vi "J-Turn.vi"(6 "Synchronication":enum16{"Start", "Wait"}(ring), 7 "Description":string, 8 "Command Info In":T2, 9 "Path Data":T1=[{"Maneuver"=enum."MAX 90", "Rotation Direction"=enum."N/A"}, {"Maneuver"=enum."MAX 90", "Rotation Direction"=enum."N/A"}, {"Maneuver"=enum."MAX 90", "Rotation Direction"=enum."N/A"}], 10 "Angle boi":dbl, 11 "Left Setpoint (Power)":dbl) -> (0 "Command Info Out":T2)   [LabVIEW 2018]
doc: "This VI notifies the subsystem to the new setpoint."
uses:
  <vilib>/Rock Robotics/WPI/Framework/Command Status Info.ctl
  <vilib>/Rock Robotics/WPI/Framework/Completion Status.ctl
  <vilib>/Rock Robotics/WPI/Framework/Completion Notifier.ctl
  Support Code/Path Data.ctl
  Implementation/Drive Operations.ctl
  Implementation/Drive Setpoints.ctl
  Support Code/Availible Command systems for auto.ctl
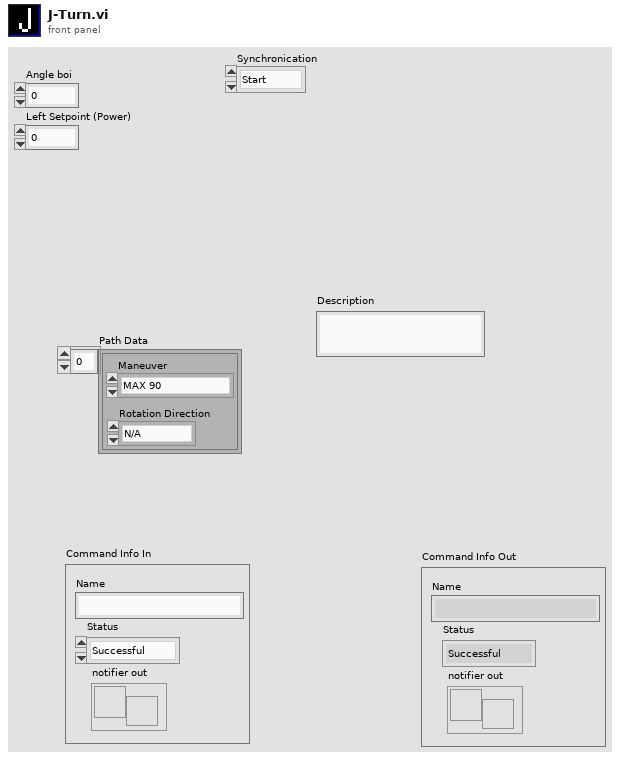
[diagram p1: front panel]
types:
  T1 = typedef "Path Data.ctl" = cluster{"Maneuver":enum16{"MAX 90", "MAX 180", "Turn to Home", "Turn to Rocket", "Auto-Align", "Turn to ..."}, "Rotation Direction":enum16{"N/A", "Right", "Left"}}[]
  T2 = typedef "Command Status Info.ctl" = cluster{"Name":string, "Status":T3, "notifier out":T4}
  T3 = typedef "Completion Status.ctl" = enum16{"Successful", "Aborted", "Incomplete"}
  T4 = typedef "Completion Notifier.ctl" = refnum<notifier>
  T5 = typedef "Drive Operations.ctl" = enum16{"Reserve", "Read Current", "Immediate", "J-Turn", "Play Back From Log", "Auto-Align"}
  T6 = typedef "Drive Setpoints.ctl" = cluster{"Operation":T5, "Left Setpoint (Power)":dbl, "Right Setpoint (Turning)":dbl, "Reverse (T) / Normal (F)":bool, "Power Scaling (1=Normal) ":dbl, "Path Data":T1, "Path":path, "Angle boi":dbl, "Path Reversed":bool, "Align for Path":bool, "80A(T)/45(F)":bool, "Auto Path Data":cluster{"V":dbl[], "Theta":dbl[], "Commands":cluster{"Time into Path":dbl, "System":T7, "Item Selected?":bool, "System Selection":T7}[], "Sample Period":dbl}}
  T7 = typedef "Availible Command systems for auto.ctl" = u16
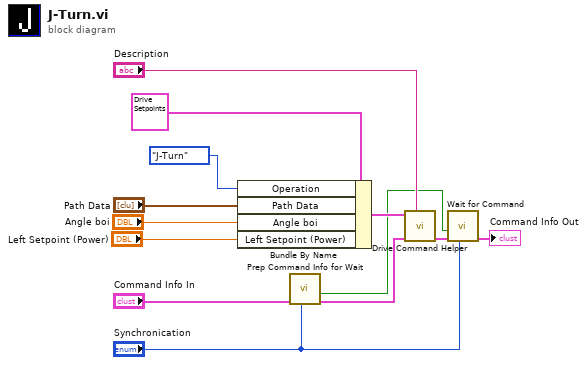
[diagram p0: block diagram]
diagram:
  n1 = Bundle By Name(cluster=T6 {"Operation"=enum."Immediate", "Left Setpoint (Power)"=0.0, "Right Setpoint (Turning)"=0.0, "Reverse (T) / Normal (F)"=FALSE, "Power Scaling (1=Normal) "=0.0, "Path Data"=[{"Maneuver"=enum."MAX 90", "Rotation Direction"=enum."N/A"}, {"Maneuver"=enum."MAX 90", "Rotation Direction"=enum."N/A"}, {"Maneuver"=enum."MAX 90", "Rotation Direction"=enum."N/A"}], "Path"=path "", "Angle boi"=0.0, "Path Reversed"=FALSE, "Align for Path"=FALSE, "80A(T)/45(F)"=FALSE, "Auto Path Data"={"V"=[], "Theta"=[], "Commands"=[], "Sample Period"=0.0}} ("SubSystem Data"), "Operation"=Drive_Operations."J-Turn", "Path Data"="Path Data", "Angle boi"="Angle boi", "Left Setpoint (Power)"="Left Setpoint (Power)") -> (w11:T6)
  n2 = call <vilib>:"Prep Command Info for Wait.vi"("Synchronication"="Synchronication", "Command Info"="Command Info In") -> ("Command Info"=w6:T2, "Allocated"=w7:bool)  [unwired: 8 in]
  n3 = call "Drive Command Helper.vi"("Description"="Description", "Command Info In"=w6, "SubSystem Data"=w11) -> ("Command Info Out"=w5:T2)  [unwired: 6 in, 2 out]
  n4 = call <vilib>:"Wait for Command.vi"("Synchronication"="Synchronication", "Command Info in"=w5, "Allocated"=w7) -> ("Command Info out"=→"Command Info Out":T2)  [unwired: 8 in]
